vi "Stoffmengen 2.2.vi"(0 "c":dbl min=0.0 max=1.0 step=0.01, 1 "h":dbl min=0.0 max=1.0 step=0.01, 2 "o":dbl min=0.0 max=1.0 step=0.01, 3 "Brennstoffmasse [g/Arbeitsspiel]":dbl, 4 "AGR- Rate":dbl(knob) min=0.01 max=0.9 step=0.01, 5 "Lambda Luft":dbl, 6 "Kammervolumen [m^3]":dbl, 7 "Hubraum [m^3]":dbl, 8 "Verdichtungsverhältnis":dbl, 9 "Anzahl Zylinder [Stück]":dbl min=0.0, 10 "Bohrungsdurchmesser [m]":dbl, 11 "exzentrität":dbl, 12 "Radius Kurbelwelle [m]":dbl, 13 "Einspritzwinkel [°]":dbl, 14 "Pleuellänge [m]":dbl) -> (16 "nO2,Kammer":dbl, 17 "nH2O,Kammer":dbl, 18 "nN2,Kammer":dbl, 19 "nCO2,Kammer":dbl, 20 "H2 [mol]":dbl, 21 "CH4 [mol]":dbl, 22 "C2H2 [mol]":dbl, 23 "O2 [mol]":dbl, 24 "N2 [mol]":dbl, 25 "Masse in Kammer [g]":dbl, 26 "Kammerumrechnungsfaktor":dbl)   [LabVIEW 2009]
uses:
  <vilib>/express/express arith-compare/Formula/XNode/ExpressFormulaBlockNode.xnode
  <vilib>/Analysis/NI_AALPro.lvlib
  <vilib>/Analysis/Matrix/NI_Matrix.lvlib
  <vilib>/Analysis/Matrix/Numeric/Conversions/Array To Matrix - RA2.vi
  <vilib>/Analysis/7linalg.llb/Solve Linear Equations (multiple right hand).vi
panel:
  in  "Molmasse C":dbl min=12.0 max=12.0
  in  "Molmasse C2H2":dbl min=26.0 max=26.0
  in  "Molmasse CH4":dbl min=16.0 max=16.0
  in  "Molmasse CO2":dbl min=44.0 max=44.0
  in  "Molmasse N2":dbl min=28.0 max=28.0
  in  "Molmasse O2":dbl min=32.0 max=32.0
  in  "Molmasse H2O":dbl min=18.0 max=18.0
  in  "Molmasse H2":dbl min=2.0 max=2.0
  # "Motorkenndaten"
  # "Molmassen [g/mol]"
  # "Verbrennungseinstellungen"
  # "Kraftstoffdaten"
  # "Optional!"
  # "Notwendig!"
  # "Ergebnisse"
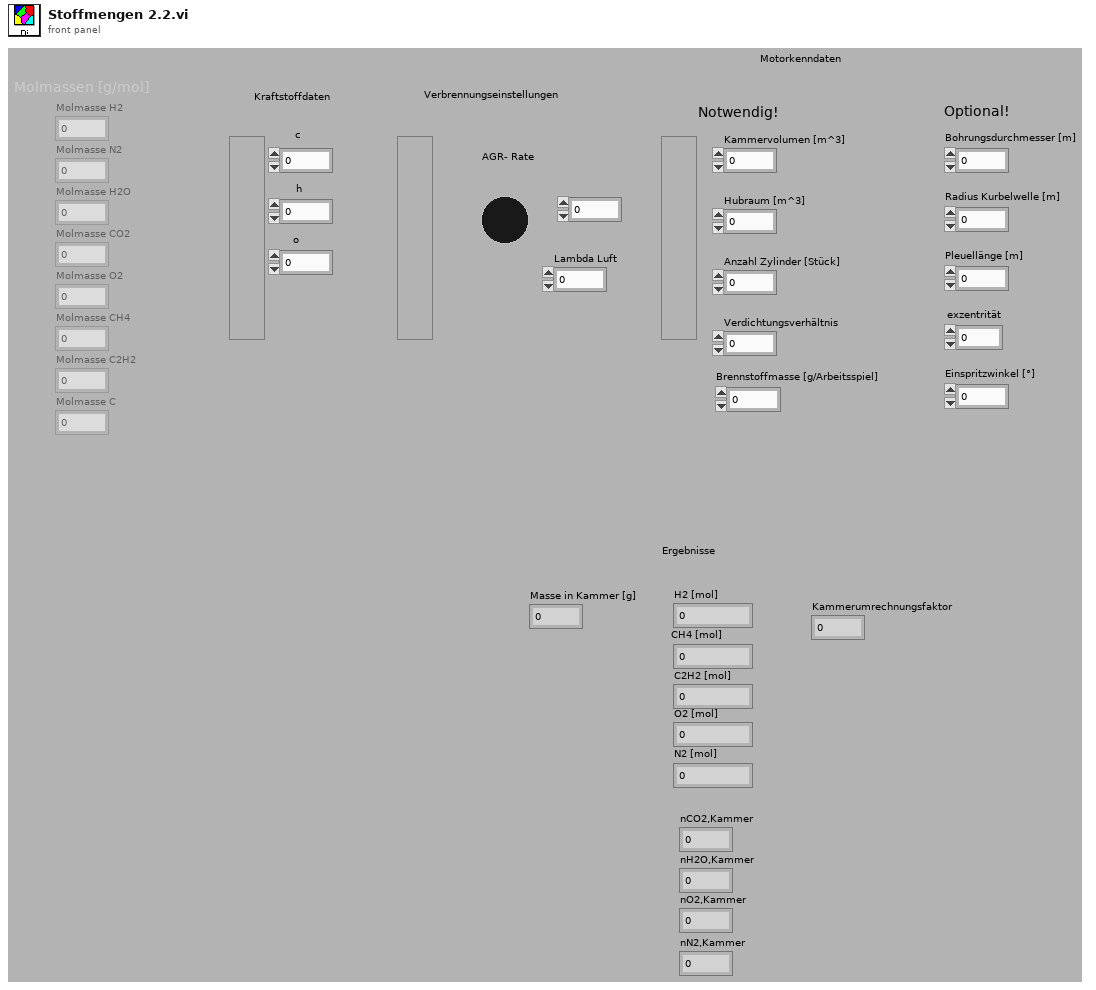
[diagram p1: front panel]
types:
  T1 = typedef "NI_Matrix.lvlib/RealMatrix.ctl" = dbl[][]
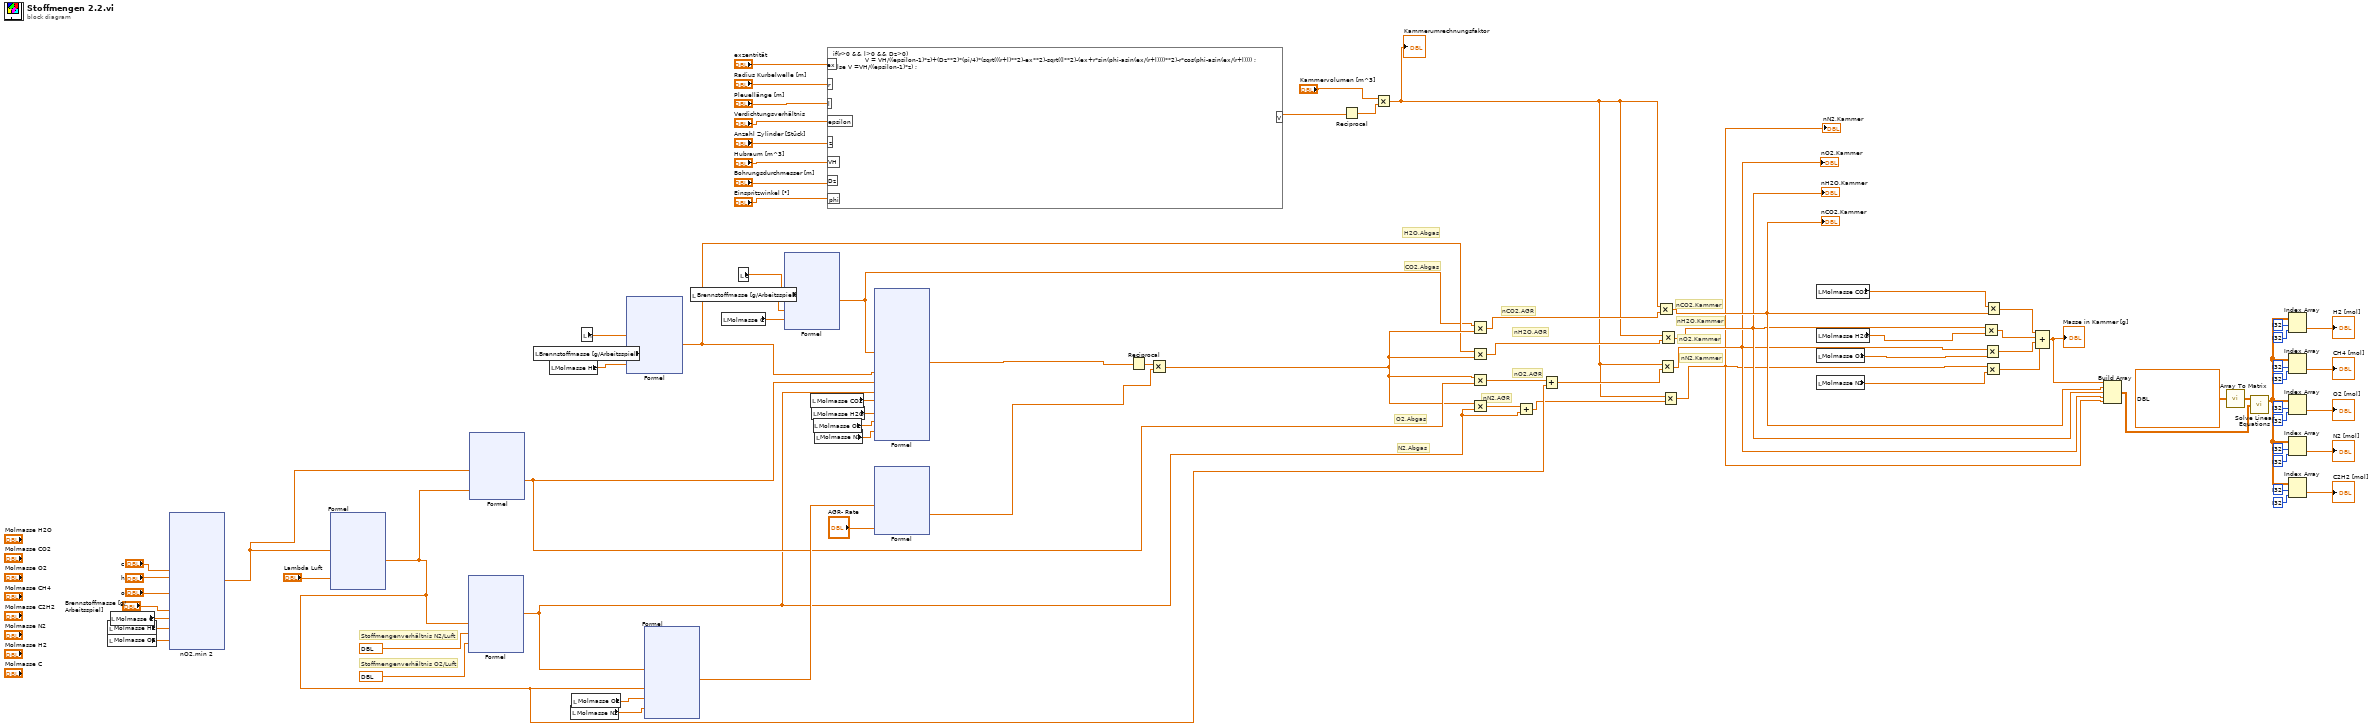
[diagram p0: block diagram]
diagram:
  # "nN2,AGR"
  # "nO2,AGR"
  # "nH2O,AGR"
  # "nCO2,AGR"
  # "nN2,Kammer"
  # "nO2,Kammer"
  # "nH2O,Kammer"
  # "nCO2,Kammer"
  # "H2O,Abgas"
  # "CO2,Abgas"
  # "O2,Abgas"
  # "N2,Abgas"
  # "Stoffmengenverhältnis O2/Luft"
  # "Stoffmengenverhältnis N2/Luft"
  n1 = local read "Molmasse H2"() -> (w30:dbl)
  n2 = local read "Molmasse O2"() -> (w29:dbl)
  n3 = local read "Molmasse C"() -> (w31:dbl)
  n4 = xnode ("nO2,min 2")("c"="c", "h"="h", "o"="o", "Brennstoffmasse"="Brennstoffmasse [g/Arbeitsspiel]", "MC"=w31, "MH2"=w30, "MO2"=w29) -> ("Ergebnis"=w22:dbl)  [unwired: 1 in, 1 out]
  n5 = xnode "Formel"("nO2min"=w22, "Lambda"="Lambda Luft") -> ("Ergebnis"=w16:dbl)  [unwired: 1 in, 1 out]
  n6 = xnode "Formel"("nO2l"=w16, "luftN2"=dbl ? ("x*y"), "luftO2"=dbl ?) -> ("Ergebnis"=w17:dbl)  [unwired: 1 in, 1 out]
  n7 = xnode "Formel"("nO2min"=w22, "nO2L"=w16) -> ("Ergebnis"=w20:dbl)  [unwired: 1 in, 1 out]
  n8 = local read "Brennstoffmasse [g/Arbeitsspiel]"() -> (w83:dbl)
  n9 = local read "Molmasse H2"() -> (w24:dbl)
  n10 = local read "Molmasse N2"() -> (w79:dbl)
  n11 = local read "Molmasse O2"() -> (w80:dbl)
  n12 = local read "h"() -> (w81:dbl)
  n13 = xnode "Formel"("h"=w81, "Brennstoffmasse"=w83, "MH2"=w24) -> ("Ergebnis"=w4:dbl)  [unwired: 1 in, 1 out]
  n14 = xnode "Formel"("nN2L"=w17, "nO2L"=w16, "MO2"=w80, "MN2"=w79) -> ("Ergebnis"=w21:dbl)  [unwired: 1 in, 1 out]
  n15 = local read "Brennstoffmasse [g/Arbeitsspiel]"() -> (w82:dbl)
  n16 = local read "Molmasse C"() -> (w25:dbl)
  n17 = local read "c"() -> (w84:dbl)
  n18 = xnode "Formel"("c"=w84, "Brennstoffmasse"=w82, "MC"=w25) -> ("Ergebnis"=w3:dbl)  [unwired: 1 in, 1 out]
  n19 = local read "Molmasse CO2"() -> (w78:dbl)
  n20 = local read "Molmasse H2O"() -> (w77:dbl)
  n21 = local read "Molmasse O2"() -> (w76:dbl)
  n22 = local read "Molmasse N2"() -> (w75:dbl)
  n23 = formula code="if(r>0 && l>0 && Dz>0)\n                V = VH/((epsilon-1)*z)+(Dz**2)*(pi/4)*(sqrt(((r+l)**2)-ex**2)-sqrt((l**2)-(ex+r*sin(phi-asin(ex/(r+l))))**2)-r*cos(phi-asin(ex/(r+l)))) ;\nelse V =VH/((epsilon-1)*z) ;"("ex"="exzentrität", "r"="Radius Kurbelwelle [m]", "l"="Pleuellänge [m]", "epsilon"="Verdichtungsverhältnis", "z"="Anzahl Zylinder [Stück]", "VH"="Hubraum [m^3]", "Dz"="Bohrungsdurchmesser [m]", "phi"="Einspritzwinkel [°]") -> ("V"=w32:dbl)
  n24 = xnode "Formel"("Luftmasse"=w21, "AGRrate"="AGR- Rate") -> ("Ergebnis"=w73:dbl)  [unwired: 1 in, 1 out]
  n25 = xnode "Formel"("nCO2abgas"=w3, "nH2Oabgas"=w4, "nO2abgas"=w20, "nN2abgas"=w17, "MCO2"=w78, "MH2O"=w77, "MO2"=w76, "MN2"=w75) -> ("Ergebnis"=w6:dbl)  [unwired: 1 in, 1 out]
  n26 = Reciprocal(x=w6) -> (1/x=w74:dbl)
  n27 = Multiply(x=w74, y=w73) -> (x*y=w5:dbl)
  n28 = Reciprocal(x=w32) -> (1/x=w72:dbl)
  n29 = Multiply(x="Kammervolumen [m^3]", y=w72) -> (x*y=w12:dbl)
  "Kammerumrechnungsfaktor" <- w12
  n30 = Multiply(x=w3, y=w5) -> (x*y=w15:dbl)
  n31 = Multiply(x=w4, y=w5) -> (x*y=w14:dbl)
  n32 = Multiply(x=w5, y=w20) -> (x*y=w18:dbl)
  n33 = Multiply(x=w5, y=w17) -> (x*y=w19:dbl)
  n34 = Add(x=w19, y=w17) -> (x+y=w11:dbl)
  n35 = Add(x=w18, y=w16) -> (x+y=w13:dbl)
  n36 = Multiply(x=w12, y=w15) -> (x*y=w10:dbl)
  "nCO2,Kammer" <- w10
  n37 = Multiply(x=w12, y=w13) -> (x*y=w8:dbl)
  "nO2,Kammer" <- w8
  n38 = Multiply(x=w12, y=w14) -> (x*y=w9:dbl)
  "nH2O,Kammer" <- w9
  n39 = Multiply(x=w12, y=w11) -> (x*y=w7:dbl)
  "nN2,Kammer" <- w7
  n40 = local read "Molmasse CO2"() -> (w71:dbl)
  n41 = local read "Molmasse H2O"() -> (w70:dbl)
  n42 = local read "Molmasse O2"() -> (w69:dbl)
  n43 = local read "Molmasse N2"() -> (w68:dbl)
  n44 = Multiply(x=w9, y=w70) -> (x*y=w66:dbl)
  n45 = Multiply(x=w8, y=w69) -> (x*y=w65:dbl)
  n46 = Multiply(x=w7, y=w68) -> (x*y=w64:dbl)
  n47 = Multiply(x=w71, y=w10) -> (x*y=w67:dbl)
  n48 = Compound Arithmetic op=ADD(w67, w66, w65, w64) -> (w46:dbl)
  "Masse in Kammer [g]" <- w46
  n49 = Build Array(w46, w10, w9, w8, w7) -> (w63:T1)
  n50 = call-poly <vilib>:"Array To Matrix.vi"("Real 2D Array"=dbl[][] ? ("Input Matrix")) -> ("Real Matrix"=w1:T1)
  n51 = call-poly <vilib>:"Solve Linear Equations.vi"("Known Matrix"=w63, "Input Matrix"=w1) -> ("Solution Matrix"=w52:T1)  [unwired: 1 in, 1 out]
  n52 = Index Array(array=w52, index (row)=i32 ? ("Index (Zeile)"), index (col)=i32 ? ("Index (Spalte)")) -> (element=→"H2 [mol]":dbl)
  n53 = Index Array(array=w52, index (row)=i32 ? ("Index (Zeile)"), index (col)=i32 ? ("Index (Spalte)")) -> (element=→"CH4 [mol]":dbl)
  n54 = Index Array(array=w52, index (row)=i32 ? ("Index (Zeile)"), index (col)=i32 ? ("Index (Spalte)")) -> (element=→"O2 [mol]":dbl)
  n55 = Index Array(array=w52, index (row)=i32 ? ("Index (Zeile)"), index (col)=i32 ? ("Index (Spalte)")) -> (element=→"N2 [mol]":dbl)
  n56 = Index Array(array=w52, index (row)=i32 ? ("Index (Zeile)"), index (col)=i32 ? ("Index (Spalte)")) -> (element=→"C2H2 [mol]":dbl)
